vi "Get Item As String.vi"(8 "error in (no error)":errorcluster, 10 "Name Array":string[](array[string]), 11 "JSON Value in":refnum<class "JSON Value.lvclass">) -> (0 "error out":errorcluster, 1 "String":string, 2 "found":bool, 3 "JSON Value out":refnum<class "JSON Value.lvclass">)   [LabVIEW 2011, in "JSON.lvlib"]
uses:
  .json-api-labview/JSON Library/JSON.lvlib
  JSON Value/JSON Value.lvclass
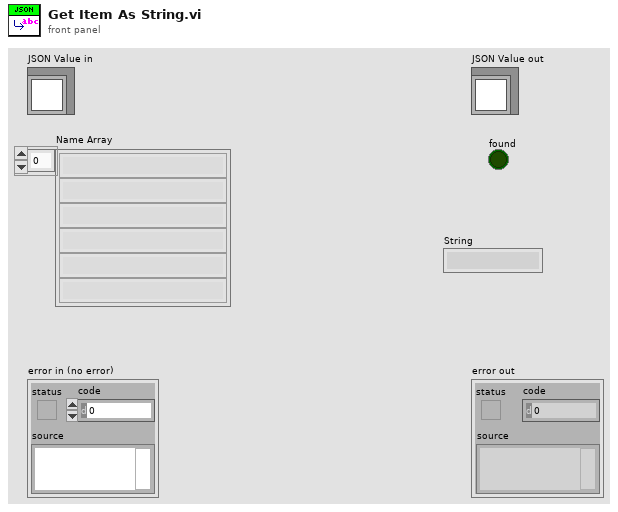
[diagram p1: front panel]
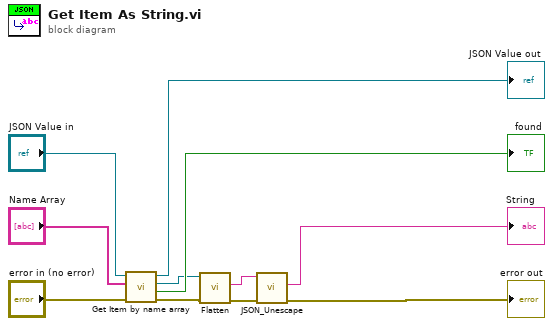
[diagram p0: block diagram]
diagram:
  n1 = call "Get Item by name array.vi"("error in (no error)"="error in (no error)", "Name Array"="Name Array", "JSON Value In"="JSON Value in") -> ("error out"=w7:errorcluster, "found"=→"found":bool, "Value"=w1:refnum<class "JSON Value.lvclass">, "JSON Value Out"=→"JSON Value out":refnum<class "JSON Value.lvclass">)  [unwired: 5 in]
  n2 = call-dynamic "Flatten.vi"("error in (no error)"=w7, "JSON Value in"=w1) -> ("error out"=w6:errorcluster, "String"=w3:string)  [unwired: 8 in]
  n3 = call "JSON_Unescape.vi"("error in (no error)"=w6, "String In"=w3) -> ("error out"=→"error out":errorcluster, "Unescaped String Out"=→"String":string)  [unwired: 7 in]
